vi "test_HostApi Byte coerced response.vi"(8 "error in (no error)":errorcluster) -> (0 "error out":errorcluster)   [LabVIEW 2019, in "Host API Tests.lvclass"]
uses:
  Host API Tests.lvclass
  Addon/Addon Shared/Types/Buffered RT Instrument Command.ctl
  Addon/Addon Shared/Types/Response Wait Type.ctl
  <vilib>/addons/_JKI Toolkits/VI Tester/TestCase.llb/TestCase.lvclass
  APIs/Host Automation API/Instrument Host Automation API.lvlib
  Addon/Addon Shared/Instrument Addon Shared.lvlib
  C:/Program Files (x86)/National Instruments/LabVIEW 2019/vi.lib/addons/_JKI Toolkits/VI Tester/TestCase.llb/TestCase.lvclass
panel:
  out "TestCase out":refnum<class "Host API Tests.lvclass">
  in  "TestCase in":refnum<class "Host API Tests.lvclass">
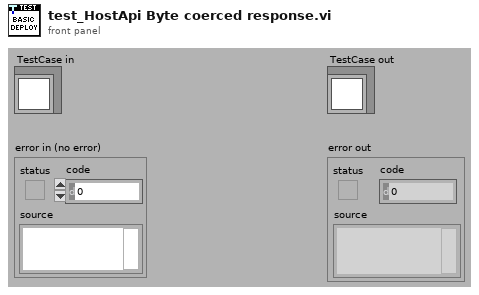
[diagram p1: front panel]
types:
  T1 = typedef "Instrument Addon Shared.lvlib/Buffered RT Instrument Command.ctl" = cluster{"Command":string, "Response Expected?":bool, "Wait Type":T2, "Wait Value":dbl}
  T2 = typedef "Instrument Addon Shared.lvlib/Response Wait Type.ctl" = enum16{"Byte Count", "Wait sec"}
  T3 = typedef "NI STM.lvlib/TCP Connection Info.ctl" = cluster{"connection ID":refnum<k5>, "meta data":T4[]}
  T4 = typedef "NI STM.lvlib/MetaDataElement.ctl" = string
  T5 = typedef "Instrument Addon Shared.lvlib/Buffered RT Instrument Request.ctl" = cluster{"Response":string, "Error":errorcluster}
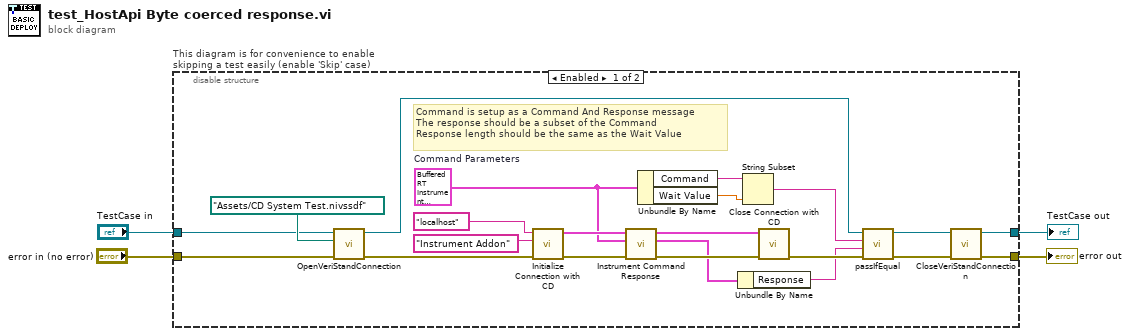
[diagram p0: block diagram]
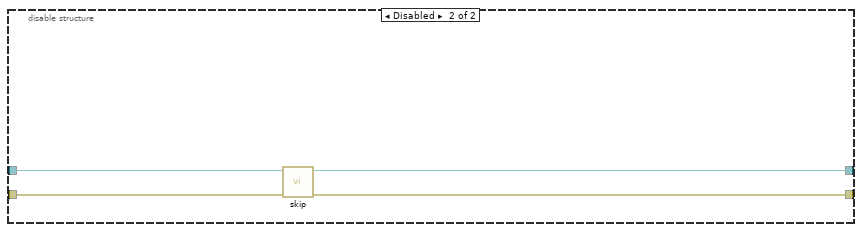
[diagram p2: hidden frame]
diagram:
  n1 = disable-structure "This diagram is for convenience to enable skipping a test easily (enable 'Skip' case)" shown="Enabled" {
    disable-tunnel: "TestCase in" -> [w22 w30]
    disable-tunnel: [w20 w28] -> w1
    disable-tunnel: [w21 w29] -> w3
    disable-tunnel: "error in (no error)" -> [w23 w27]
    frame Enabled {
      w10 = T1 {"Command"="15CommandResponse", "Response Expected?"=TRUE, "Wait Type"=enum."Byte Count", "Wait Value"=10.0}  # Command Parameters
      # "Command is setup as a Command And Response message\nThe response should be a subset of the Command\nResponse length should be the same as the Wait Value"
      n2 = call-dynamic "OpenVeriStandConnection.vi"("error in (no error)"=w23, "System Definition File"=path "Assets/CD System Test.nivssdf", "VeriStand Test Case in"=w22) -> ("error out"=w19:errorcluster, "VeriStand Test Case out"=w12:refnum<class "Host API Tests.lvclass">)  [unwired: 6 in, 1 out]
      n3 = call "Initialize Connection with CD.vi"("error in (no error)"=w19, "TCP Service"="Instrument Addon", "IP Address"="localhost") -> ("error out"=w16:errorcluster, "connection info out"=w11:T3)  [unwired: 7 in]
      n4 = call "Instrument Command Response.vi"("error in (no error)"=w16, "Command Parameters"=w10, "Comm.Info"=w11) -> ("error out"=w14:errorcluster, "Response"=w9:T5, "Comm.Info"=w13:T3)  [unwired: 5 in, 1 out]
      n5 = Unbundle By Name(w10) -> ("Command"=w7:string, "Wait Value"=w6:dbl)
      n6 = Unbundle By Name(w9) -> ("Response"=w8:string)
      n7 = String Subset(string=w7, length (rest)=w6) -> (substring=w5:string)  [unwired: 1 in]
      n8 = call "Close Connection with CD.vi"("error in"=w14, "Comm.Info"=w13) -> ("error out"=w15:errorcluster)  [unwired: 9 in]
      n9 = call-dynamic "passIfEqual.vi"("error in (no error)"=w15, "y"=w8, "x"=w5, "TestCase in"=w12) -> ("error out"=w18:errorcluster, "TestCase out"=w17:refnum<class "Host API Tests.lvclass">)  [unwired: 6 in]
      n10 = call-dynamic "CloseVeriStandConnection.vi"("error in (no error)"=w18, "VeriStand Test Case in"=w17) -> ("error out"=w21:errorcluster, "VeriStand Test Case out"=w20:refnum<class "Host API Tests.lvclass">)  [unwired: 8 in]
    }
    frame Disabled {
      # "skip test result while test is under development"
      n11 = call <vilib>:"skip.vi"("error in (no error)"=w27, "TestCase in"=w30) -> ("error out"=w29:errorcluster, "TestCase out"=w28:refnum<class "Host API Tests.lvclass">)  [unwired: 8 in]
    }
  }
  "error out" <- w3
  "TestCase out" <- w1
